vi "readBoolean.vi"(8 "error in (no error)":errorcluster, 11 "ModbusTriggerControl in":refnum<class "ModbusTriggerControl.lvclass">) -> (0 "error out":errorcluster, 2 "Data":bool, 3 "IBoolean out":refnum<class "ModbusTriggerControl.lvclass">)   [LabVIEW 2016, in "ModbusTriggerControl.lvclass"]
uses:
  ModbusTriggerControl.lvclass
  ModbusTriggerControl.lvclass/ModbusTriggerControl.ctl
  FPGA/FPGA.lvclass
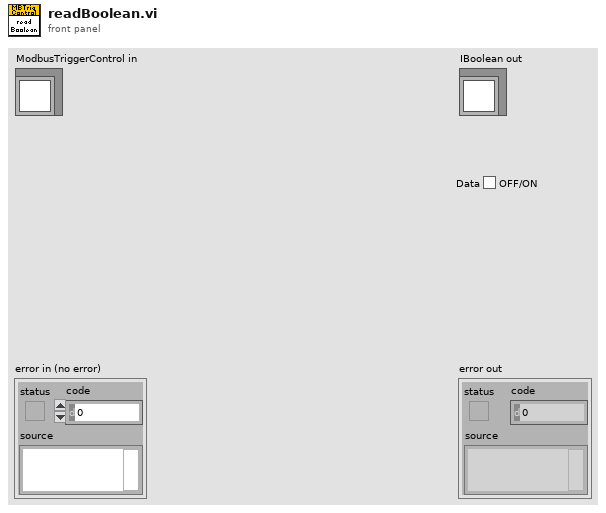
[diagram p1: front panel]
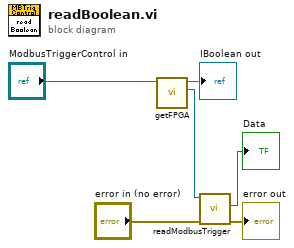
[diagram p0: block diagram]
diagram:
  n1 = call "getFPGA.vi"("ModbusTriggerControl in"="ModbusTriggerControl in") -> ("FPGA"=w4:refnum<class "FPGA.lvclass">, "ModbusTriggerControl out"=→"IBoolean out":refnum<class "ModbusTriggerControl.lvclass">)  [unwired: 9 in]
  n2 = call "readModbusTrigger.vi"("error in (no error)"="error in (no error)", "FPGA in"=w4) -> ("error out"=→"error out":errorcluster, "Trigger"=→"Data":bool)  [unwired: 7 in, 1 out]
